vi "PrepareFileForLoadll.vi"(0 "indexed loaded Array":dbl[][](array[numeric]), 3 "Nickname":string, 4 "Min":dbl, 5 "Max":dbl, 6 "Index":i32, 7 "Load Value Name Array":string[](array[string]), 8 "Display Message":bool, 9 "Load Value Array":dbl[](array[numeric])) -> (14 "indexed loaded Array":dbl[][](array[numeric]), 18 "Successful?":bool)   [LabVIEW 2014, in "Panels.lvlib"]
uses:
  Panels.lvlib
  Instance           1 28Saved   PrepareFileForLoadll .vi
  Instance           2 28Saved   PrepareFileForLoadll .vi
panel:
  in  "No Link?":bool
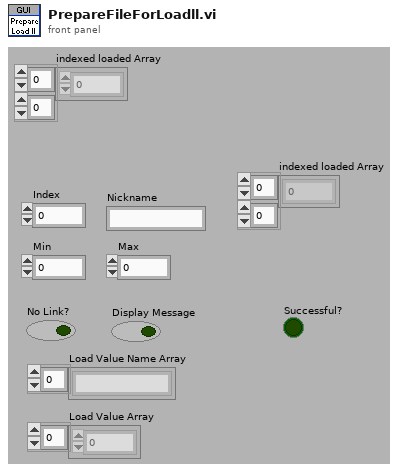
[diagram p1: front panel]
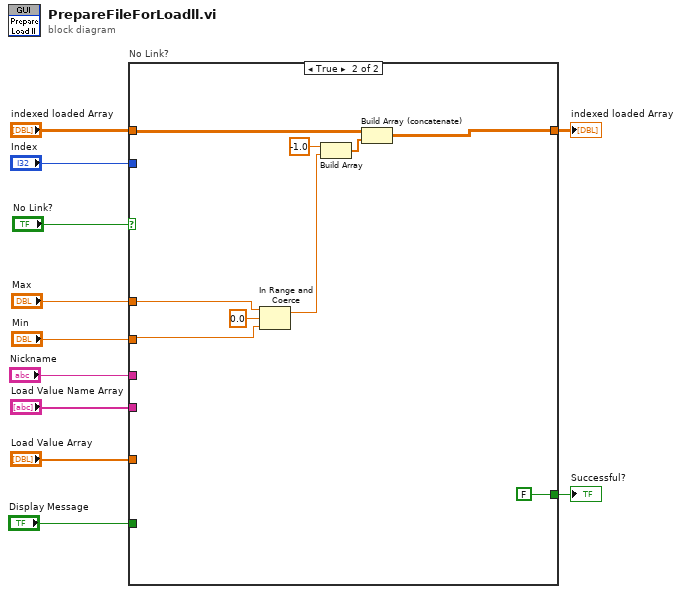
[diagram p0: block diagram]
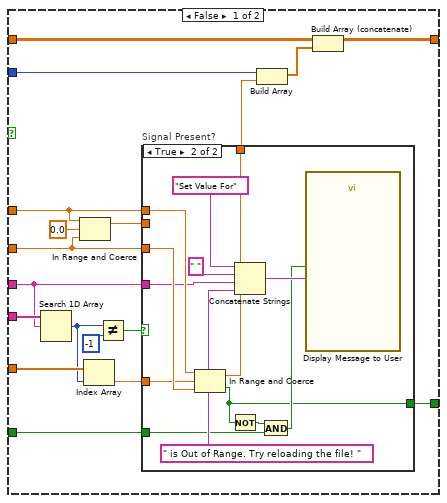
[diagram p2: hidden frame]
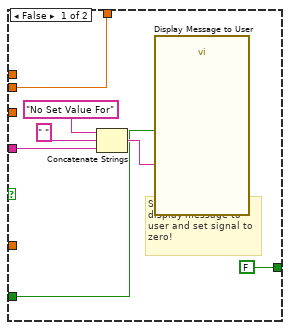
[diagram p3: hidden frame]
diagram:
  n1 = case "No Link?" shown="True" "No Link?" {
    tunnel: "Nickname" -> [w27 _]
    tunnel: "Load Value Name Array" -> [w29 _]
    tunnel: "Load Value Array" -> [w25 _]
    tunnel: [w20 w55] -> w10
    tunnel: "Display Message" -> [w22 _]
    tunnel: "Min" -> [w14 w52]
    tunnel: "Max" -> [w15 w53]
    tunnel: "Index" -> [w21 _]
    tunnel: "indexed loaded Array" -> [w19 w57]
    tunnel: [w12 FALSE] -> w1
    frame False {
      n2 = Search 1D Array(1D array=w29, element=w27) -> (index of element=w24:i32)  [unwired: 1 in]
      n3 = In Range and Coerce(upper limit=w15, x=0.0, lower limit=w14) -> (coerced(x)=w13:dbl)  [unwired: 1 out]
      n4 = Index Array(array=w25, index=w24) -> (element=w17:dbl)
      n5 = Not Equal?(x=w24, y=-1) -> (x != y?=w26:bool)
      n6 = case "Signal Present?" shown="True" w26 {
        tunnel: [w31 w49] -> w23
        tunnel: w27 -> [w35 w43]
        tunnel: w22 -> [w32 w39]
        tunnel: w14 -> [_ w48]
        tunnel: w15 -> [_ w47]
        tunnel: w17 -> [_ w41]
        tunnel: w13 -> [w31 _]
        tunnel: [FALSE w37] -> w12
        frame False {
          # "Signal is not present display message to user and set signal to zero!"
          n7 = Concatenate Strings("No Set Value For" ("Message"), " " ("string"), w35) -> (w33:string)
          n8 = call "Display Message to User"("Enable"=w32, "Message"=w33) -> ()  [unwired: 8 in, 2 out]
        }
        frame True {
          n9 = In Range and Coerce(upper limit=w47, x=w41, lower limit=w48) -> (coerced(x)=w49:dbl, In Range?=w37:bool)
          n10 = Not(x=w37) -> (.not. x?=w38:bool)
          n11 = Concatenate Strings("Set Value For" ("Message"), " " ("string"), w43, " is Out of Range. Try reloading the file! " ("Message")) -> (w44:string)
          n12 = And(x=w38, y=w39) -> (x .and. y?=w40:bool)
          n13 = call "Display Message to User"("Enable"=w40, "Message"=w44) -> ()  [unwired: 8 in, 2 out]
        }
      }
      n14 = Build Array(w21, w23) -> (w18:dbl[])
      n15 = Build Array (concatenate)(w19, w18) -> (w20:dbl[][])
    }
    frame True {
      n16 = In Range and Coerce(upper limit=w53, x=0.0, lower limit=w52) -> (coerced(x)=w51:dbl)  [unwired: 1 out]
      n17 = Build Array(-1.0 ("element"), w51) -> (w56:dbl[])
      n18 = Build Array (concatenate)(w57, w56) -> (w55:dbl[][])
    }
  }
  "indexed loaded Array" <- w10
  "Successful?" <- w1
